vi "Get Attribute VAR.vi"(8 "error in":errorcluster, 10 "Attribute":string, 11 "IConfigurable in":refnum<class "IConfigurable.lvclass">) -> (0 "error out":errorcluster, 2 "Value":variant, 3 "IConfigurable out":refnum<class "IConfigurable.lvclass">)   [LabVIEW 2024, in "IConfigurable.lvclass"]
uses:
  IConfigurable.lvclass
  IConfigure/IConfigure.lvclass
  IConfiguration/IConfiguration.lvclass
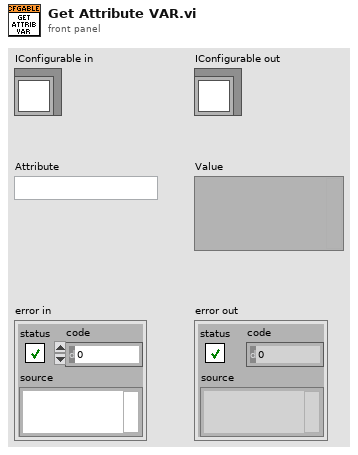
[diagram p1: front panel]
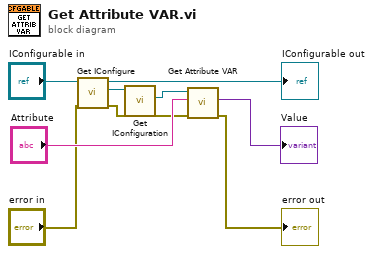
[diagram p0: block diagram]
diagram:
  n1 = call-dynamic "Get IConfigure.vi"("error in"="error in", "IConfigurable in"="IConfigurable in") -> ("error out"=w3:errorcluster, "IConfigure"=w7:refnum<class "IConfigure.lvclass">, "IConfigurable out"=→"IConfigurable out":refnum<class "IConfigurable.lvclass">)  [unwired: 7 in]
  n2 = call-dynamic "Get IConfiguration.vi"("IConfigure in"=w7) -> ("IConfiguration"=w1:refnum<class "IConfiguration.lvclass">)  [unwired: 9 in, 1 out]
  n3 = call-dynamic "Get Attribute VAR.vi"("error in"=w3, "Attribute"="Attribute", "IConfiguration in"=w1) -> ("error out"=→"error out":errorcluster, "Value"=→"Value":variant)  [unwired: 6 in, 1 out]
